vi "数码显示.vi"(11 "数值":i32) -> (2 "Cluster":T1 caption="簇")   [LabVIEW 2024]
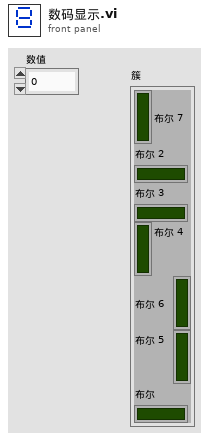
[diagram p1: front panel]
types:
  T1 = cluster{"布尔 7":bool, "布尔 2":bool, "布尔 3":bool, "布尔 4":bool, "布尔 6":bool, "布尔 5":bool, "布尔":bool}
  T2 = cluster{"[0]":bool, "[1]":bool, "[2]":bool, "[3]":bool, "[4]":bool, "[5]":bool, "[6]":bool}
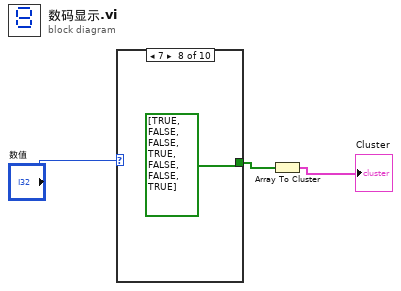
[diagram p0: block diagram]
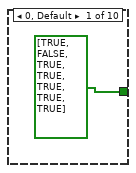
[diagram p2: hidden frame]
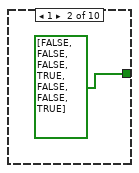
[diagram p3: hidden frame]
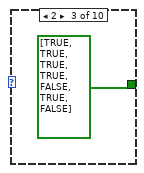
[diagram p4: hidden frame]
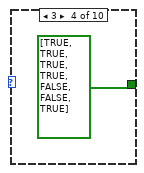
[diagram p5: hidden frame]
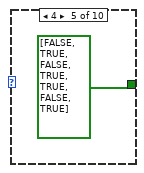
[diagram p6: hidden frame]
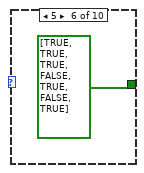
[diagram p7: hidden frame]
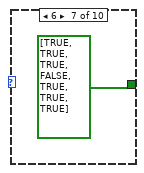
[diagram p8: hidden frame]
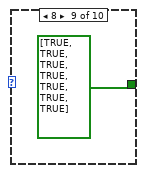
[diagram p9: hidden frame]
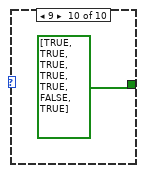
[diagram p10: hidden frame]
diagram:
  n1 = case shown="7" "数值" {
    tunnel: [bool[] [TRUE, FALSE, TRUE, TRUE, TRUE, TRUE, TRUE] bool[] [FALSE, FALSE, FALSE, TRUE, FALSE, FALSE, TRUE] bool[] [TRUE, TRUE, TRUE, TRUE, FALSE, TRUE, FALSE] bool[] [TRUE, TRUE, TRUE, TRUE, FALSE, FALSE, TRUE] bool[] [FALSE, TRUE, FALSE, TRUE, TRUE, FALSE, TRUE] bool[] [TRUE, TRUE, TRUE, FALSE, TRUE, FALSE, TRUE] bool[] [TRUE, TRUE, TRUE, FALSE, TRUE, TRUE, TRUE] bool[] [TRUE, FALSE, FALSE, TRUE, FALSE, FALSE, TRUE] bool[] [TRUE, TRUE, TRUE, TRUE, TRUE, TRUE, TRUE] bool[] [TRUE, TRUE, TRUE, TRUE, TRUE, FALSE, TRUE]] -> w2
    frame 0, Default {
    }
    frame 1 {
    }
    frame 2 {
    }
    frame 3 {
    }
    frame 4 {
    }
    frame 5 {
    }
    frame 6 {
    }
    frame 7 {
    }
    frame 8 {
    }
    frame 9 {
    }
  }
  n2 = Array To Cluster(array=w2) -> (cluster=→"Cluster":T2)
